vi "Get Data Notifier.vi"(8 "error in (no error)":errorcluster, 10 "Name":string, 11 "Task Base in":refnum<class "Task Base.lvclass">) -> (0 "error out":errorcluster, 2 "Data Notifier":refnum<notifier>, 3 "Task Base out":refnum<class "Task Base.lvclass">)   [LabVIEW 2023, in "HAL GOOP4.lvlib" / "Task Base.lvclass"]
uses:
  Task Base.lvclass
  Task Base.lvclass/Task Base.ctl
  <vilib>/ErrorRing/Error Ring.xnode
  <vilib>/Utility/error.llb/Error Cluster From Error Code.vi
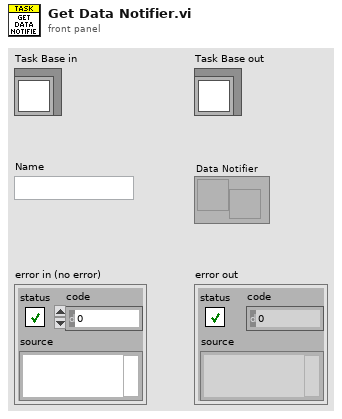
[diagram p1: front panel]
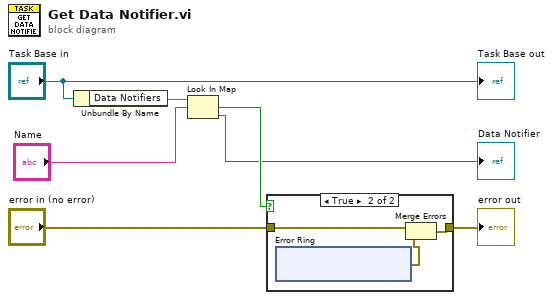
[diagram p0: block diagram]
diagram:
  n1 = Unbundle By Name("Task Base in") -> ("Data Notifiers"=w6:map{string, refnum<notifier>})
  n2 = Look In Map(map=w6, key="Name") -> (key not found?=w3:bool, value=→"Data Notifier":refnum<notifier>)  [unwired: 1 in]
  n3 = case shown="True" w3 {
    tunnel: "error in (no error)" -> [w8 w11]
    tunnel: [w8 w10] -> w1
    frame False {
    }
    frame True {
      n4 = xnode "Error Ring"() -> ("error out"=w9:errorcluster)
      n5 = Merge Errors(w11, w9) -> (w10:errorcluster)
    }
  }
  "error out" <- w1
  "Task Base out" <- "Task Base in"
